vi "ShowTestView.vi"(8 "error in (no error)":errorcluster, 9 "Floating":bool=TRUE, 11 "reference in":refnum<class "Test_Template.lvclass">) -> (0 "error out":errorcluster, 2 "UI":refnum<vi>, 3 "reference in":refnum<class "Test_Template.lvclass">)   [LabVIEW 2017]
uses:
  Test_Template.lvclass
  Components/TestView_Base.lvlibp/TestView_Base.lvclass
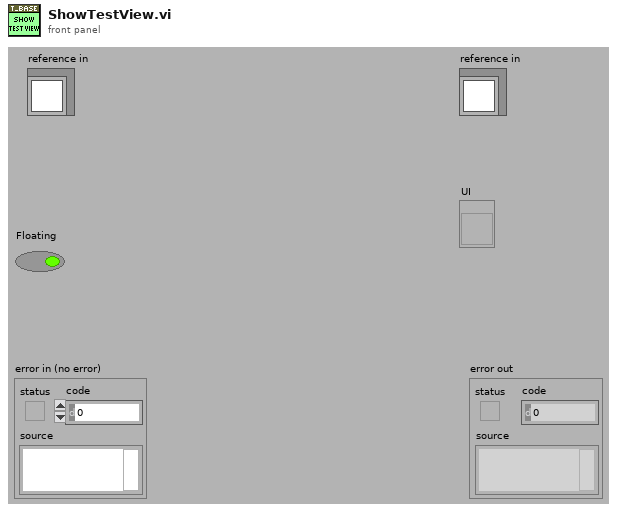
[diagram p1: front panel]
types:
  T1 = typedef "Test_Template.lvlib/Test_Template.lvclass/ObjectAttributes.ctl" = cluster{"Config":T2}
  T2 = typedef "Test_Template.lvlib/Test_Template.lvclass/Config.ctl" = cluster{"default":string}
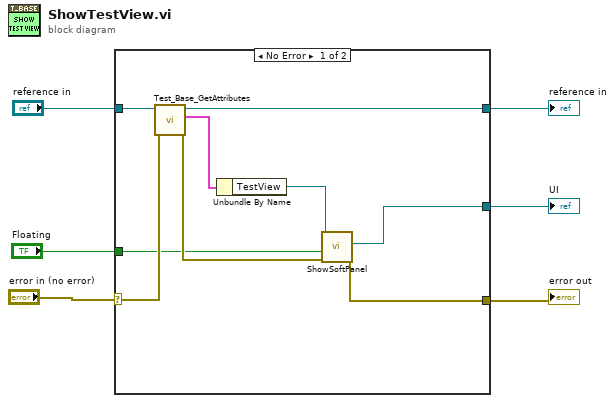
[diagram p0: block diagram]
diagram:
  n1 = case shown="No Error" "error in (no error)" {
    selector: "error in (no error)" -> [w15 w17]
    tunnel: [w9 w17] -> w5
    tunnel: [w12 w16] -> w3
    tunnel: "reference in" -> [w13 w16]
    tunnel: "Floating" -> [w8 _]
    tunnel: [w7 _] -> w1
    frame No Error {
      n2 = call "Test_Base_GetAttributes.vi"("error in (no error)"=w15, "reference in"=w13) -> ("error out"=w10:errorcluster, "Data"=w14:T1, "reference out"=w12:refnum<class "Test_Template.lvclass">)  [unwired: 6 in, 1 out]
      n3 = Unbundle By Name(w14) -> ("TestView"=w11:refnum<class "TestView_Base.lvclass">)
      n4 = call-dynamic "ShowSoftPanel.vi"("error in (no error)"=w10, "Floating"=w8, "Driver in"=w11) -> ("error out"=w9:errorcluster, "vi reference"=w7:refnum<vi>)  [unwired: 6 in, 1 out]
    }
    frame Error {
    }
  }
  "error out" <- w5
  "reference in" <- w3
  "UI" <- w1
